vi "Send reply (SubVI).vi"(5 "return_msg":string, 6 "Correlation ID":string, 7 "retcode":u16(ring) items=["0"=0, "1"=1, "100"=100, "101"=101, "102"=102, "200"=200, "201"=202, "300"=300, "301"=301, "302"=302, "303"=303, "304"=304, "305"=305, "306"=306, "307"=307, "308"=308, "309"=309, "400"=400, "500"=500, "501"=501, "502"=502, "999"=999], 8 "error in (no error)":errorcluster, 9 "reply content":string, 10 "target":string, 11 "Exchange.lvclass":refnum<class "Exchange.lvclass">) -> (0 "error out":errorcluster, 2 "sent message":string)   [LabVIEW 2016]
uses:
  <vilib>/Distrio/LabbitMQ/Exchange/Exchange.lvclass
panel:
  out "Exchange out":refnum<class "Exchange.lvclass">
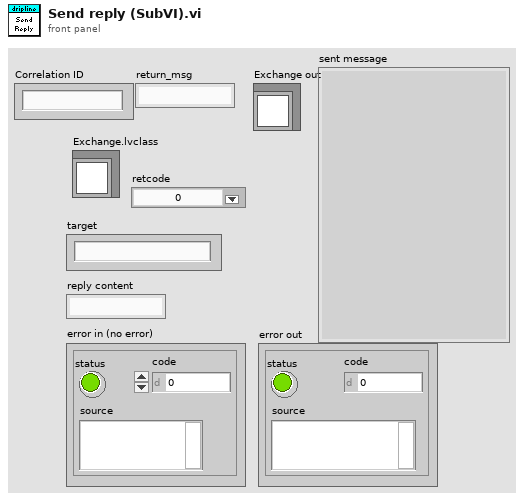
[diagram p1: front panel]
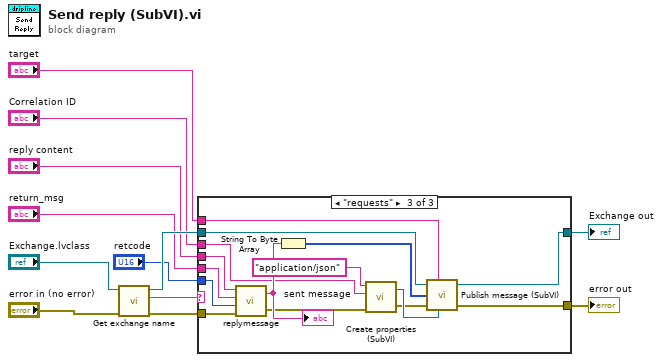
[diagram p0: block diagram]
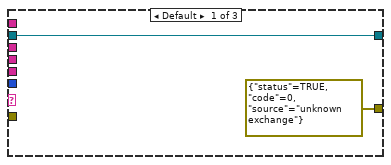
[diagram p2: hidden frame]
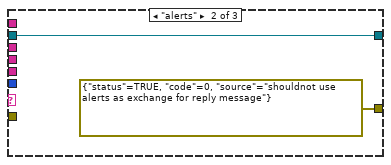
[diagram p3: hidden frame]
diagram:
  n1 = call <vilib>:"Get exchange name.vi"("error in (no error)"="error in (no error)", "Exchange in"="Exchange.lvclass") -> ("error out"=w12:errorcluster, "name"=w8:string, "Exchange out"=w10:refnum<class "Exchange.lvclass">)  [unwired: 7 in]
  n2 = case shown="\"requests\"" w8 {
    tunnel: w12 -> [_ _ w31]
    tunnel: w10 -> [w13 w15 w22]
    tunnel: "target" -> [_ _ w25]
    tunnel: [errorcluster {"status"=TRUE, "code"=0, "source"="unknown exchange"} ("error constant") errorcluster {"status"=TRUE, "code"=0, "source"="shouldnot use alerts as exchange for reply message"} ("error constant") w17] -> w6
    tunnel: "reply content" -> [_ _ w30]
    tunnel: "Correlation ID" -> [_ _ w23]
    tunnel: [w13 w15 w21] -> w3
    tunnel: "return_msg" -> [_ _ w20]
    tunnel: "retcode" -> [_ _ w19]
    frame Default {
    }
    frame "alerts" {
    }
    frame "requests" {
      n3 = call "replymessage.vi"("error in (no error)"=w31, "retcode"=w19, "return_msg"=w20, "reply content"=w30) -> ("error out"=w18:errorcluster, "body"=w24:string)
      "sent message" <- w24
      n4 = String To Byte Array(string=w24) -> (unsigned byte array=w28:u8[])
      n5 = call "Create properties (SubVI).vi"("error in (no error)"=w18, "CorrelationId"=w23, "ContentEncoding"="application/json") -> ("error out"=w26:errorcluster, "reference out"=w27:refnum<k24>)  [unwired: 1 in]
      n6 = call "Publish message (SubVI).vi"("Exchange in"=w22, "target"=w25, "body"=w28, "error in (no error)"=w26, "MessageProperties"=w27) -> ("Exchange out"=w21:refnum<class "Exchange.lvclass">, "error out"=w17:errorcluster)  [unwired: 1 in]
    }
  }
  "error out" <- w6
  "Exchange out" <- w3
